vi "TicWriteTest.vi"() -> ()   [LabVIEW 2021]
panel:
  in  "Address":u16=16384 caption="Address [16384=Unadressed]" max=16384
  out "Time(s)":dbl
  out "target(mm)":i32
  in  "Pulses/mm":i32=400
  out "TotalDistance(m)":dbl format="%.2f"
  out "Loops":i32
  in  "readInterval(ms)":u32=100
  out "target(pulses)":i32
  in  "interMoveDelayMax(s)":dbl=5.0
  in  "moveTimeout(s)":dbl=60.0
  in  "VISA resource name":refnum<visa-resource-name>="ASRL1::INSTR"
  in  "Stop Button":bool
  in  "Max(mm)":i32=250
  out "Position(pulses)":i32
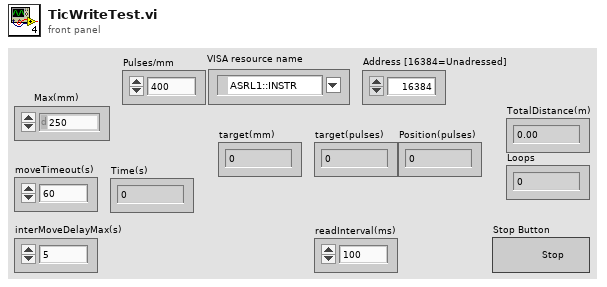
[diagram p1: front panel]
types:
  T1 = enum16{"GetStatus", "GetPosition", "SetTarget", "Enable", "Disable", "SetCurrent", "GetVelocity", "GetUptime", "GetVsupply", "Reset", "Go"}
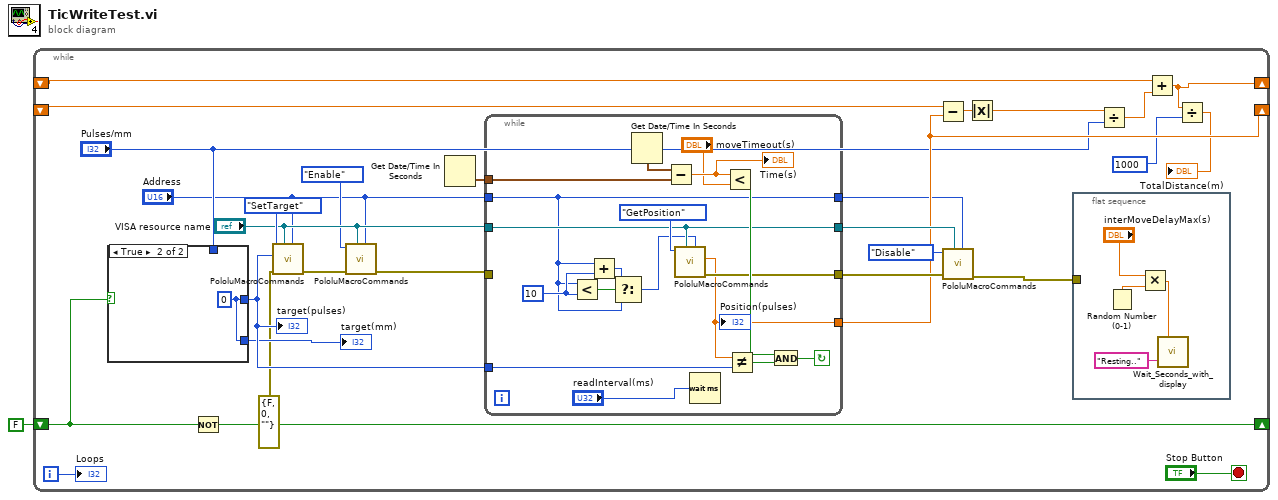
[diagram p0: block diagram]
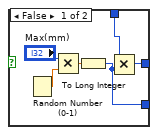
[diagram p2: hidden frame]
diagram:
  n1 = while {
    shift-right: [w18] -> _
    shift-left: FALSE -> [w19]
    shift-right: [w14] -> _
    shift-left: _ -> [w15]
    shift-right: [w12] -> _
    shift-left: _ -> [w11]
    i -> [w17]
    stop <- "Stop Button" stop-if-true
    n2 = case shown="True" w19 {
      tunnel: [w33 w37] -> w16
      tunnel: "Pulses/mm" -> [w32 _]
      tunnel: [w31 w37] -> w5
      frame False {
        n3 = Random Number (0-1)() -> (number: 0 to 1=w35:dbl)
        n4 = Multiply(x="Max(mm)", y=w35) -> (x*y=w34:dbl)
        n5 = To Long Integer(number=w34) -> (32bit integer=w31:i32)
        n6 = Multiply(x=w32, y=w31) -> (x*y=w33:i32)
      }
      frame True {
        w37 = 0
      }
    }
    "target(pulses)" <- w16
    "target(mm)" <- w5
    n7 = Not(x=w19) -> (.not. x?=w18:bool)
    n8 = call "PololuMacroCommands.vi"("Address"="Address", "Port Name (VISA)"="VISA resource name", "Error In"=errorcluster {"status"=FALSE, "code"=0, "source"=""}, "Argument"=w16, "Procedure"=T1."SetTarget" ("Enum")) -> ("Error Out"=w22:errorcluster)  [unwired: 4 in, 2 out]
    n9 = call "PololuMacroCommands.vi"("Address"="Address", "Port Name (VISA)"="VISA resource name", "Error In"=w22, "Procedure"=T1."Enable" ("Enum")) -> ("Error Out"=w23:errorcluster)  [unwired: 5 in, 2 out]
    n10 = Get Date/Time In Seconds() -> (seconds since 1Jan1904=w28:timestamp)
    n11 = while {
      tunnel: w23 -> [_]
      tunnel: "VISA resource name" -> [w48]
      tunnel: w16 -> [w57]
      tunnel: w28 -> [w55]
      tunnel: [w50] -> w27
      tunnel: [w48] -> w24
      tunnel: [w47] -> w12
      tunnel: "Address" -> [w43]
      tunnel: [w43] -> w3
      stop <- w52 continue-if-true
      w46 = u16 10 ("y")
      n12 = Less?(x=w43, y=w46) -> (x < y?=w45:bool)
      n13 = Add(x=w43, y=w46) -> (x+y=w44:u16)
      n14 = Select(t=w44, s=w45, f=w43) -> (s? t:f=w42:u16)
      n15 = Get Date/Time In Seconds() -> (seconds since 1Jan1904=w56:timestamp)
      n16 = Subtract(x=w56, y=w55) -> (x-y=w54:dbl)
      "Time(s)" <- w54
      n17 = call "PololuMacroCommands.vi"("Address"=w42, "Port Name (VISA)"=w48, "Procedure"=T1."GetPosition" ("Enum")) -> ("Error Out"=w50:errorcluster, "Scaled Readback"=w47:dbl)  [unwired: 6 in, 1 out]
      "Position(pulses)" <- w47
      n18 = Wait (ms)(milliseconds to wait="readInterval(ms)") -> ()  [unwired: 1 out]
      n19 = Less?(x=w54, y="moveTimeout(s)") -> (x < y?=w51:bool)
      n20 = Not Equal?(x=w47, y=w57) -> (x != y?=w59:bool)
      n21 = And(x=w51, y=w59) -> (x .and. y?=w52:bool)
    }
    n22 = Subtract(x=w11, y=w12) -> (x-y=w10:dbl)
    n23 = call "PololuMacroCommands.vi"("Address"=w3, "Port Name (VISA)"=w24, "Error In"=w27, "Procedure"=T1."Disable" ("Enum")) -> ("Error Out"=w26:errorcluster)  [unwired: 5 in, 2 out]
    n24 = Absolute Value(x=w10) -> (abs(x)=w9:dbl)
    n25 = flat-sequence {
      tunnel: w26 -> [_]
      frame #0 {
        n26 = Random Number (0-1)() -> (number: 0 to 1=w41:dbl)
        n27 = Multiply(x="interMoveDelayMax(s)", y=w41) -> (x*y=w40:dbl)
        n28 = call "Wait_Seconds_with_display.vi"("Message"="Resting..", "Seconds to wait"=w40) -> ()  [unwired: 1 in, 1 out]
      }
    }
    n29 = Divide(x=w9, y="Pulses/mm") -> (x/y=w13:dbl)
    n30 = Add(x=w15, y=w13) -> (x+y=w14:dbl)
    n31 = Divide(x=w14, y=1000 ("x")) -> (x/y=→"TotalDistance(m)":dbl)
    "Loops" <- w17
  }
